vi "test Filtering Changed Items.vi"(8 "error in":errorcluster, 11 "TestCase in":refnum<class "Refresh.lvclass">) -> (0 "error out":errorcluster, 3 "TestCase out":refnum<class "Refresh.lvclass">)   [LabVIEW 2020, in "Refresh.lvclass"]
uses:
  Refresh.lvclass
  System Explorer/Implementation/System Explorer/Refresh/MCL Row.ctl
  System Explorer/Implementation/System Explorer/Refresh/Change Type.ctl
  System Explorer/Implementation/System Explorer/Refresh/Symbols.ctl
  <vilib>/addons/_JKI Toolkits/VI Tester/TestCase.llb/TestCase.lvclass
  System Explorer/Implementation/System Explorer/Refresh/Refresh.lvlib
  C:/Program Files (x86)/National Instruments/LabVIEW 2020/vi.lib/addons/_JKI Toolkits/VI Tester/TestCase.llb/TestCase.lvclass
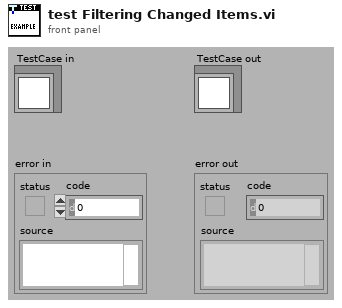
[diagram p1: front panel]
types:
  T1 = typedef "AIM MIL-STD-1553 System Explorer.lvlib/Implementation.lvlib/Refresh.lvlib/MCL Row.ctl" = cluster{"change type":T2, "item symbol":T3, "item names":string[]}
  T2 = typedef "AIM MIL-STD-1553 System Explorer.lvlib/Implementation.lvlib/Refresh.lvlib/Change Type.ctl" = enum16{"No change", "Modify", "Add", "Remove"}
  T3 = typedef "AIM MIL-STD-1553 System Explorer.lvlib/Implementation.lvlib/Refresh.lvlib/Symbols.ctl" = enum16{"Blank", "MIL-STD-1553", "Port", "Remote Terminal", "Subaddress", "Bus Controller", "Frame", "Mode Code", "Message", "Parameter", "Item"}
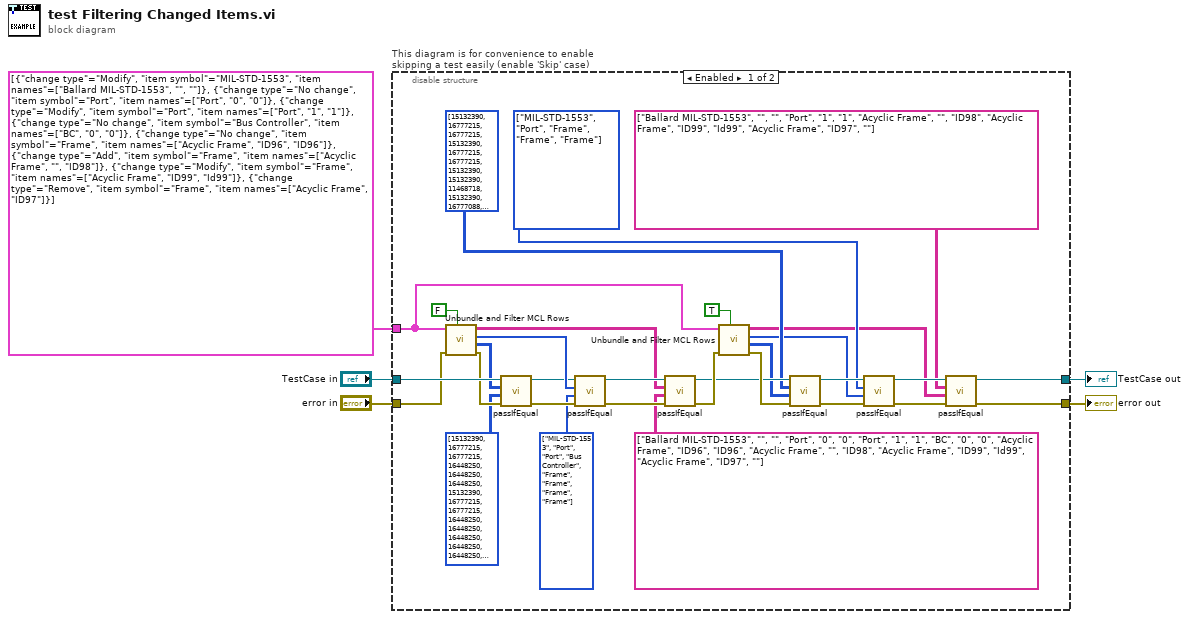
[diagram p0: block diagram]
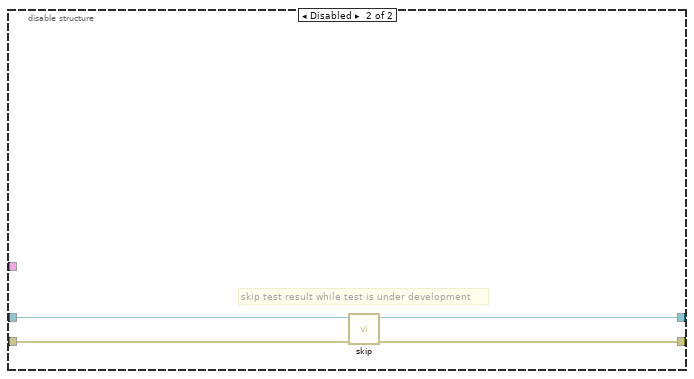
[diagram p2: hidden frame]
diagram:
  n1 = disable-structure "This diagram is for convenience to enable skipping a test easily (enable 'Skip' case)" shown="Enabled" {
    disable-tunnel: "TestCase in" -> [w29 w40]
    disable-tunnel: [w14 w38] -> w2
    disable-tunnel: [w13 w39] -> w4
    disable-tunnel: "error in" -> [w27 w37]
    disable-tunnel: T1[] [{"change type"=enum."Modify", "item symbol"=enum."MIL-STD-1553", "item names"=["Ballard MIL-STD-1553", "", ""]}, {"change type"=enum."No change", "item symbol"=enum."Port", "item names"=["Port", "0", "0"]}, {"change type"=enum."Modify", "item symbol"=enum."Port", "item names"=["Port", "1", "1"]}, {"change type"=enum."No change", "item symbol"=enum."Bus Controller", "item names"=["BC", "0", "0"]}, {"change type"=enum."No change", "item symbol"=enum."Frame", "item names"=["Acyclic Frame", "ID96", "ID96"]}, {"change type"=enum."Add", "item symbol"=enum."Frame", "item names"=["Acyclic Frame", "", "ID98"]}, {"change type"=enum."Modify", "item symbol"=enum."Frame", "item names"=["Acyclic Frame", "ID99", "Id99"]}, {"change type"=enum."Remove", "item symbol"=enum."Frame", "item names"=["Acyclic Frame", "ID97"]}] ("refresh items in") -> [w6 _]
    frame Enabled {
      w10 = T3[] [enum."MIL-STD-1553", enum."Port", enum."Frame", enum."Frame", enum."Frame"] items=["Blank", "MIL-STD-1553", "Port", "Remote Terminal", "Subaddress", "Bus Controller", "Frame", "Mode Code", "Message", "Parameter", "Item"] ("item symbols")
      w26 = T3[] [enum."MIL-STD-1553", enum."Port", enum."Port", enum."Bus Controller", enum."Frame", enum."Frame", enum."Frame", enum."Frame"] items=["Blank", "MIL-STD-1553", "Port", "Remote Terminal", "Subaddress", "Bus Controller", "Frame", "Mode Code", "Message", "Parameter", "Item"] ("item symbols")
      n2 = call "Unbundle and Filter MCL Rows.vi"("filter changed items"=FALSE, "error in"=w27, "refresh items"=w6) -> ("error out"=w28:errorcluster, "background colors"=w23:u32[][], "item symbols"=w33:T3[], "item names"=w34:string[][])  [unwired: 5 in]
      n3 = call-dynamic "passIfEqual.vi"("error in (no error)"=w28, "y"=u32[][] [[15132390, 16777215, 16777215], [16448250, 16448250, 16448250], [15132390, 16777215, 16777215], [16448250, 16448250, 16448250], [16448250, 16448250, 16448250], [15132390, 15132390, 11468718], [15132390, 16777088, 16777088], [15132390, 16761281, 15132390]], "x"=w23, "TestCase in"=w29) -> ("error out"=w30:errorcluster, "TestCase out"=w31:refnum<class "Refresh.lvclass">)  [unwired: 6 in]
      n4 = call-dynamic "passIfEqual.vi"("error in (no error)"=w30, "y"=w26, "x"=w33, "TestCase in"=w31) -> ("error out"=w35:errorcluster, "TestCase out"=w36:refnum<class "Refresh.lvclass">)  [unwired: 6 in]
      n5 = call-dynamic "passIfEqual.vi"("error in (no error)"=w35, "y"=string[][] [["Ballard MIL-STD-1553", "", ""], ["Port", "0", "0"], ["Port", "1", "1"], ["BC", "0", "0"], ["Acyclic Frame", "ID96", "ID96"], ["Acyclic Frame", "", "ID98"], ["Acyclic Frame", "ID99", "Id99"], ["Acyclic Frame", "ID97", ""]] ("item names"), "x"=w34, "TestCase in"=w36) -> ("error out"=w16:errorcluster, "TestCase out"=w15:refnum<class "Refresh.lvclass">)  [unwired: 6 in]
      n6 = call "Unbundle and Filter MCL Rows.vi"("filter changed items"=TRUE, "error in"=w16, "refresh items"=w6) -> ("error out"=w22:errorcluster, "background colors"=w12:u32[][], "item symbols"=w9:T3[], "item names"=w8:string[][])  [unwired: 5 in]
      n7 = call-dynamic "passIfEqual.vi"("error in (no error)"=w22, "y"=w12, "x"=u32[][] [[15132390, 16777215, 16777215], [15132390, 16777215, 16777215], [15132390, 15132390, 11468718], [15132390, 16777088, 16777088], [15132390, 16761281, 15132390]], "TestCase in"=w15) -> ("error out"=w21:errorcluster, "TestCase out"=w20:refnum<class "Refresh.lvclass">)  [unwired: 6 in]
      n8 = call-dynamic "passIfEqual.vi"("error in (no error)"=w21, "y"=w9, "x"=w10, "TestCase in"=w20) -> ("error out"=w18:errorcluster, "TestCase out"=w17:refnum<class "Refresh.lvclass">)  [unwired: 6 in]
      n9 = call-dynamic "passIfEqual.vi"("error in (no error)"=w18, "y"=w8, "x"=string[][] [["Ballard MIL-STD-1553", "", ""], ["Port", "1", "1"], ["Acyclic Frame", "", "ID98"], ["Acyclic Frame", "ID99", "Id99"], ["Acyclic Frame", "ID97", ""]] ("item names"), "TestCase in"=w17) -> ("error out"=w13:errorcluster, "TestCase out"=w14:refnum<class "Refresh.lvclass">)  [unwired: 6 in]
    }
    frame Disabled {
      # "skip test result while test is under development"
      n10 = call <vilib>:"skip.vi"("error in (no error)"=w37, "TestCase in"=w40) -> ("error out"=w39:errorcluster, "TestCase out"=w38:refnum<class "Refresh.lvclass">)  [unwired: 8 in]
    }
  }
  "error out" <- w4
  "TestCase out" <- w2
